vi "reshapeAndExtract.vi"(9 "window":T2={"2^n : x"=10, "2^n : y"=10, "lower left box Position"={"X"=1752.0, "Y"=1167.0}, "Height"=0, "Width"=0} {"Width" min=32 max=4704; "Height" min=2 max=3424; "2^n : y" min=1 max=13; "2^n : x" min=1 max=13}, 11 "output array":u16[][](array[numeric])) -> (3 "subarray":dbl[][](array[numeric]))   [LabVIEW 2018, in "Photon Filtering.lvlib"]
uses:
  Photon Filtering.lvlib
  <vilib>/Utility/miscctls.llb/LVPointDoubleTypeDef.ctl
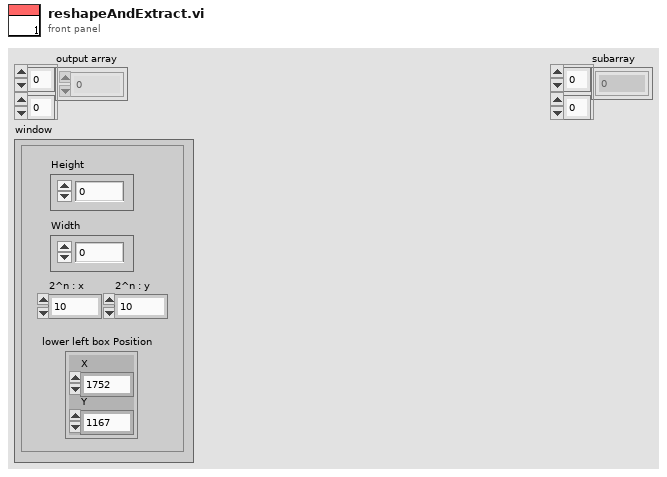
[diagram p1: front panel]
types:
  T1 = typedef "LVPointDoubleTypeDef.ctl" = cluster{"X":dbl, "Y":dbl}
  T2 = cluster{"2^n : x":i8, "2^n : y":i8, "lower left box Position":T1, "Height":i32, "Width":i32}
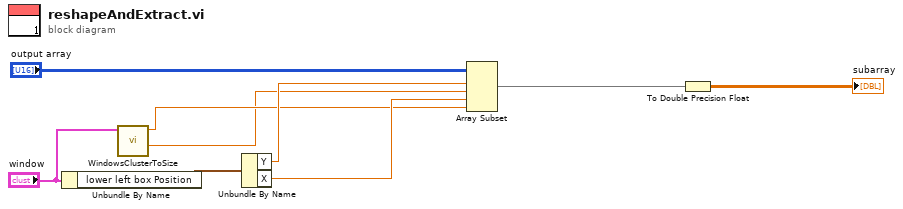
[diagram p0: block diagram]
diagram:
  n1 = Unbundle By Name("window") -> ("lower left box Position"=w8:T1)
  n2 = call "WindowsClusterToSize.vi"("subwindow control 2"="window") -> ("Ny"=w3:dbl, "Nx"=w4:dbl)  [unwired: 9 in]
  n3 = Unbundle By Name(w8) -> ("Y"=w7:dbl, "X"=w6:dbl)
  n4 = Array Subset(array="output array", index (row)=w7, length (row)=w3, index (col)=w6, length (col)=w4) -> (w2:u16[][])
  n5 = To Double Precision Float(number=w2) -> (double precision float=→"subarray":dbl[][])
